vi "Delta_Hz.vi"(1 "Counts":u32) -> (0 "Delta":u32)   [LabVIEW 2014]
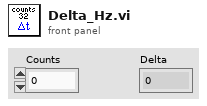
[diagram p1: front panel]
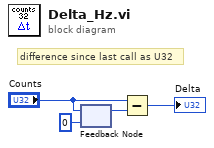
[diagram p0: block diagram]
diagram:
  # "difference since last call as U32"
  n1 = feedback-in #1("Counts") -> ()
  n2 = feedback #1(u32 0 ("element")) -> (w4:u32)
  n3 = Subtract(x="Counts", y=w4) -> (x-y=→"Delta":u32)
